vi "Main.vi"() -> ()   [LabVIEW 2025]
doc: "This template is for the Queued Message Handler design pattern.\n\nThe Event Handling Loop generates messages based on user interface actions.\n\nThe Message Handling Loop processes messages generated by the Event Handling Loop, or by other messages. The messages are string values, so new messages can be added easily to the Message Cases case structure in the Message Handling Loop. Each message cluster can also provide an optional value for Message Data, which is a variant that can be converted to whatever message-specific data is required."
uses:
  controls/UI Data.ctl
  support/Message Queue/Enqueue Message (Single).vi
  config/Stop Parse.vi
  <vilib>/Utility/error.llb/Error Cluster From Error Code.vi
  <vilib>/ErrorRing/Error Ring.xnode
  support/Message Queue/Message Queue.lvlib
  support/User Event - Stop/User Event - Stop.lvlib
panel:
  in  "CSV config sections":string[](array[string])=["RAW", "BESTXYZ", "TIME", "PSRDOP", "HWMONITOR", "GPGSV"]
  in  "OEM719 Log Parser":enum32{"OEM719 Log Parser", "Prompt"}(tab)
  in  "Stop Parse Btn":bool
  in  "Start Parse Btn":bool
  out "Notifications":string
  in  "Exit":bool
  in  "OEM 719 Simulated Log":path
  in  "offset (in bytes) (1000000)":i64=1000000
  in  "Duration (s)":dbl=30.0
  out "Elapsed_time":dbl format="%<%H:%M:%S%2u>t"
  in  "CSV File Names":string[](array[string])=["GPS RAW DATA.csv", "BESTXYZ.csv", "GPS TIME.csv", "GPS PSRDOP.csv", "GPS HWMONITOR.csv", "GPS GPGSV.csv"]
  out "Array":path[](array[path])
  # "OEM 719 Log Parser"
  # "Develop a LabVIEW application in a project to parse the provided “OEM719 Simulated Log.txt” data into separate .csv files for each distinct message type.\n•\tThe script should capture data at a frequency of 1 Hz for a duration of 30 seconds. \n•\tParsing the “OEM719 Simulated Log.txt” file should begin from an offset of 1000000 bytes from the start of the file or when the GPS acquires lock.\n•\t Each .csv file should include headers as specified in the OEM719 manual or see “GPS Logs Solution” for reference. \n•\tDo not modify the OEM719 Simulated Log.txt file."
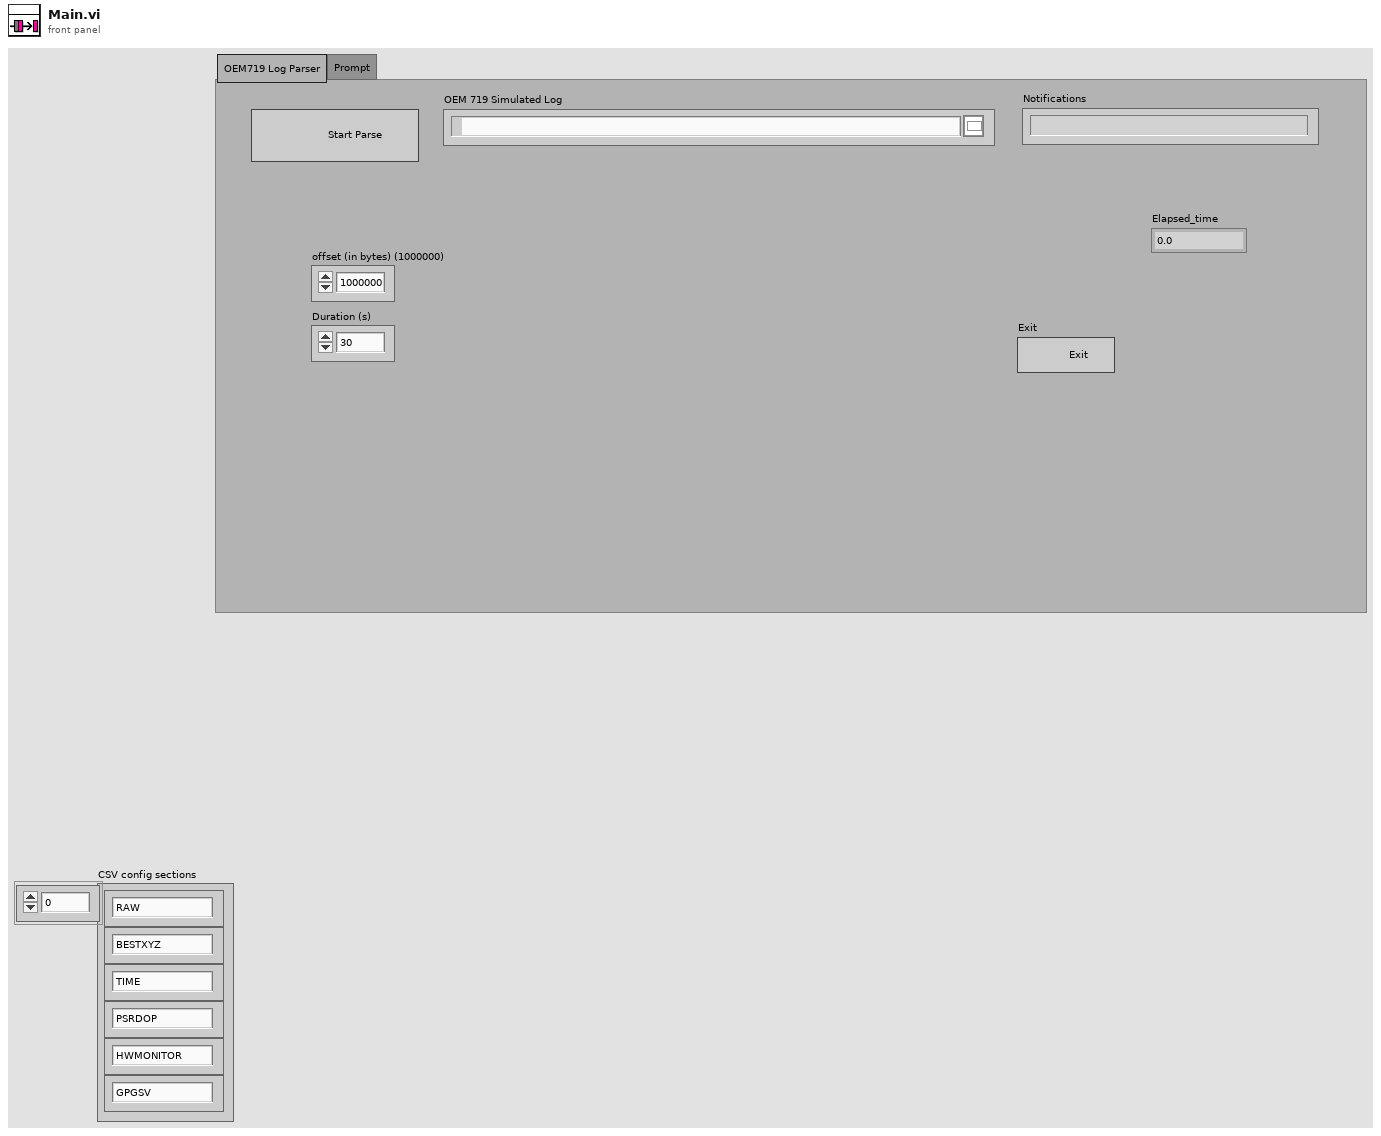
[diagram p1: front panel]
types:
  T1 = typedef "UI Data.ctl" = cluster{"Initialize Btn Ref":refnum<vi>, "Start Parse":refnum<vi>, "Data Display Ref":refnum<vi>, "Exit Button Ref":refnum<vi>}
  T2 = typedef "Message Queue.lvlib/All Message Queues.ctl" = cluster{"UI":refnum<queue>}
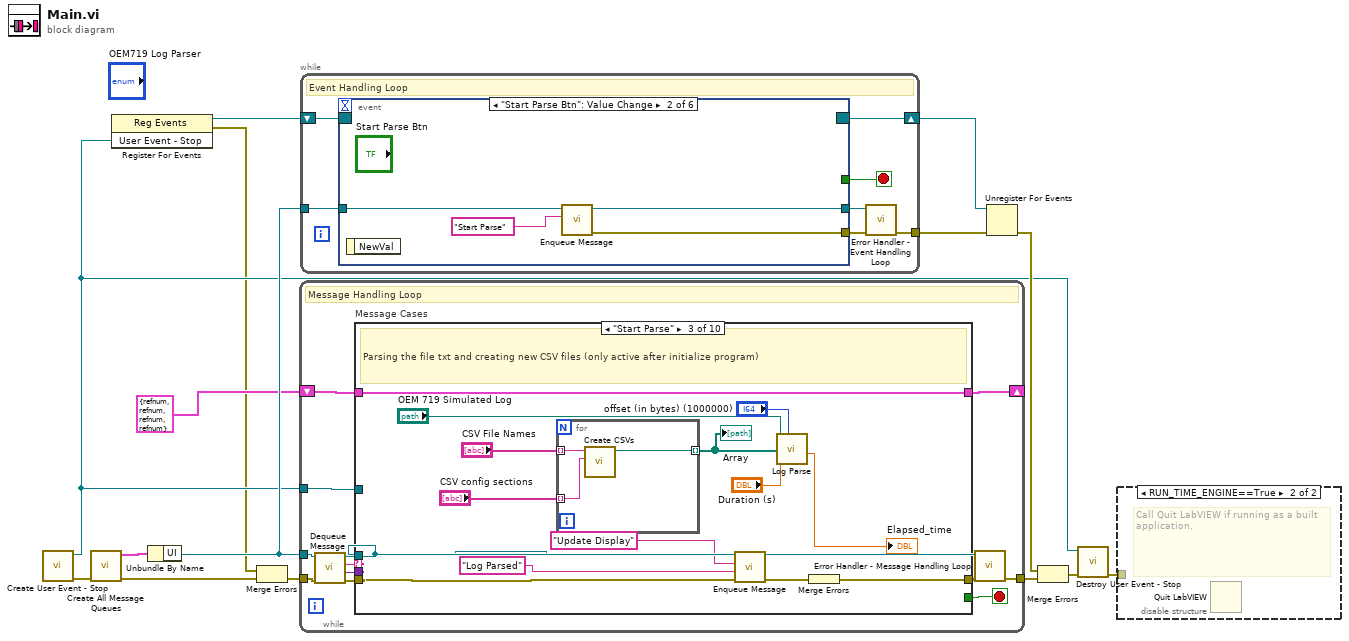
[diagram p0: block diagram]
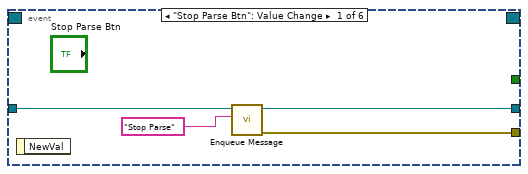
[diagram p3: hidden frame]
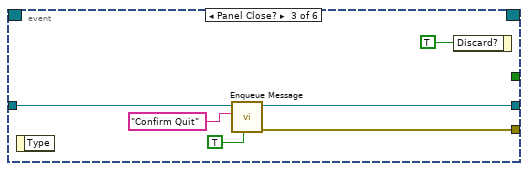
[diagram p4: hidden frame]
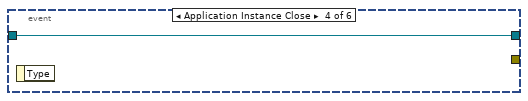
[diagram p5: hidden frame]
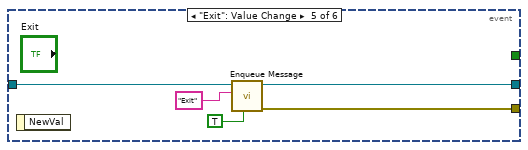
[diagram p6: hidden frame]
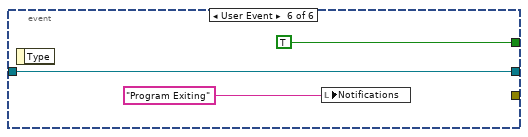
[diagram p7: hidden frame]
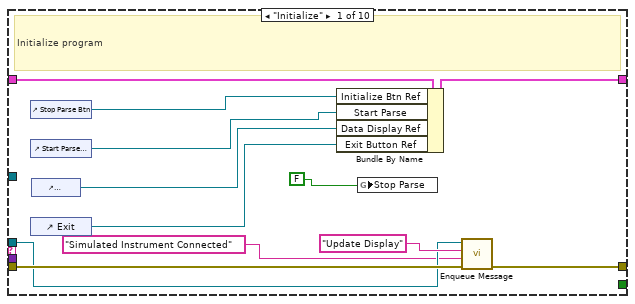
[diagram p8: hidden frame]
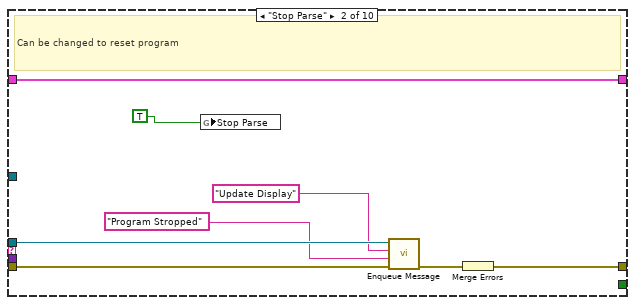
[diagram p9: hidden frame]
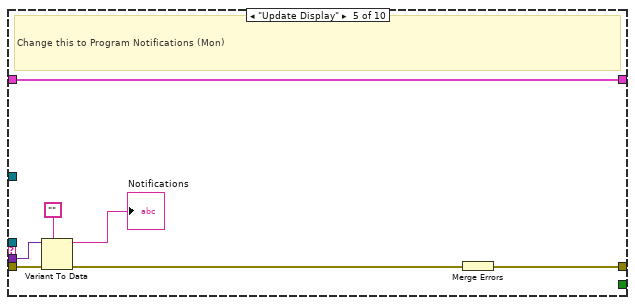
[diagram p11: hidden frame]
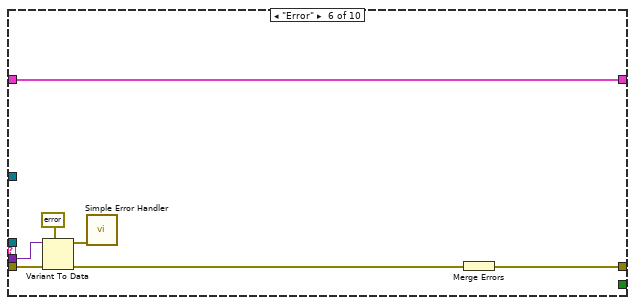
[diagram p12: hidden frame]
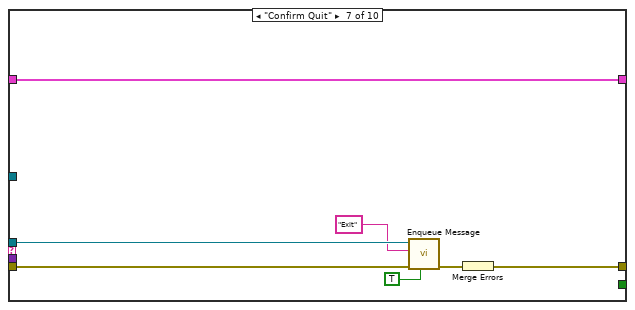
[diagram p13: hidden frame]
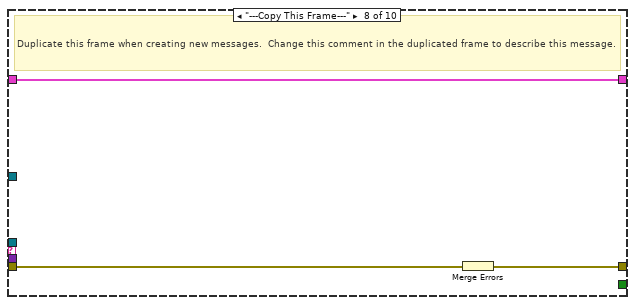
[diagram p14: hidden frame]
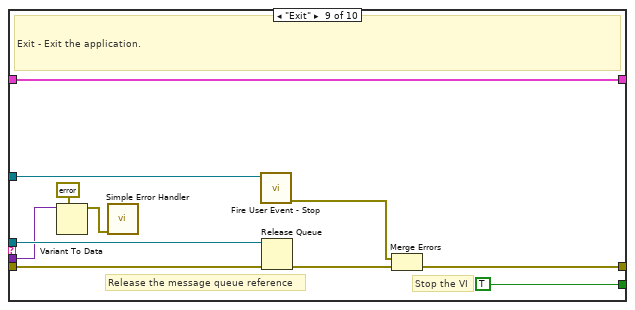
[diagram p15: hidden frame]
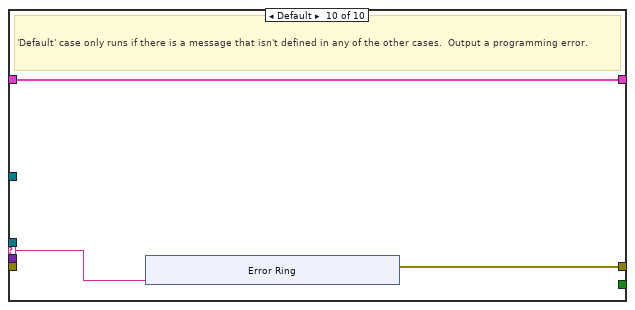
[diagram p16: hidden frame]
diagram:
  n1 = call "Create User Event - Stop.vi"() -> ("error out"=w11:errorcluster, "User Event - Stop"=w3:refnum<user-event>)  [unwired: 10 in]
  n2 = call "Create All Message Queues.vi"("error in (no error)"=w11) -> ("error out"=w15:errorcluster, "Message Queues out"=w14:T2)  [unwired: 9 in]
  n3 = register-events(w3) -> (reference out=w4:refnum<event-registration>, error out=w1:errorcluster)  [unwired: 2 in]
  n4 = Unbundle By Name(w14) -> ("UI"=w12:refnum<queue>)
  n5 = Merge Errors(w1, w15) -> (w2:errorcluster)
  n6 = while {
    tunnel: w12 -> [w19]
    shift-right: [w26] -> _
    shift-left: T1 {"Initialize Btn Ref"=refnum, "Start Parse"=refnum, "Data Display Ref"=refnum, "Exit Button Ref"=refnum} ("Data Cluster") -> [w27]
    tunnel: w3 -> [w24]
    tunnel: w2 -> [w23]
    tunnel: [w17] -> w13
    stop <- w25 stop-if-true
    # "Message Handling Loop"
    n7 = call "Dequeue Message.vi"("error in (no error)"=w23, "Message Queue"=w19) -> ("error out"=w22:errorcluster, "Message Data"=w20:variant, "Message"=w21:string, "dup Message Queue"=w18:refnum<queue>)  [unwired: 6 in]
    n8 = case "Message Cases" shown="\"Start Parse\"" w21 {
      selector: w21 -> [_ _ _ _ _ _ _ _ _ w102]
      tunnel: w18 -> [w31 w43 w50 _ _ _ w83 _ w101 _]
      tunnel: w22 -> [w38 w45 w49 w66 w71 w80 w87 w90 w94 _]
      tunnel: [w39 w46 w60 w66 w72 w74 w85 w88 w97 w103] -> w16
      tunnel: w27 -> [w37 w47 w61 w65 w73 w79 w86 w89 w100 w104]
      tunnel: [w36 w47 w61 w65 w73 w79 w86 w89 w100 w104] -> w26
      tunnel: [_ _ _ _ _ _ _ _ TRUE _] -> w25
      tunnel: w20 -> [_ _ _ _ w70 w78 _ _ w91 _]
      tunnel: w24 -> [_ _ _ _ _ _ _ _ w96 _]
      frame "Initialize" {
        # "Initialize program"
        n9 = control-ref of="Stop Parse Btn"() -> (w35:refnum<vi>)
        n10 = control-ref of="Start Parse Btn"() -> (w29:refnum<vi>)
        n11 = control-ref of="Exit"() -> (w33:refnum<vi>)
        n12 = control-ref of="Notifications"() -> (w34:refnum<vi>)
        n13 = Bundle By Name(cluster=w37, "Initialize Btn Ref"=w35, "Start Parse"=w29, "Data Display Ref"=w34, "Exit Button Ref"=w33) -> (w36:T1)
        n14 = global write "Stop Parse.vi" "Stop Parse"(FALSE) -> ()
        n15 = call-poly "Enqueue Message.vi"("error in (no error)"=w38, "Message Data"="Simulated Instrument Connected" ("Initial Message"), "Message"="Update Display", "Message Queue"=w31) -> ("error out"=w39:errorcluster)  [unwired: 6 in, 1 out]
      }
      frame "Stop Parse" {
        # "Can be changed to reset program"
        n16 = global write "Stop Parse.vi" "Stop Parse"(TRUE) -> ()
        n17 = call-poly "Enqueue Message.vi"("error in (no error)"=w45, "Message Data"="Program Stropped" ("\"Do Something\" button pressed"), "Message"="Update Display", "Message Queue"=w43) -> ("error out"=w44:errorcluster)  [unwired: 6 in, 1 out]
        n18 = Merge Errors(w44) -> (w46:errorcluster)
      }
      frame "Start Parse" {
        # "Parsing the file txt and creating new CSV files (only active after initialize program)"
        n19 = for {
          tunnel: "CSV File Names" -> [w64] mode=indexing
          tunnel: "CSV config sections" -> [w63] mode=indexing
          tunnel: [w62] -> w54 mode=indexing
          n20 = call "Create CSVs.vi"("CSV config section"=w63, "CSV File Name"=w64) -> ("CSV refnum"=w62:path)  [unwired: 8 in, 1 out]
        }
        "Array" <- w54
        n21 = call-poly "Enqueue Message.vi"("error in (no error)"=w49, "Message Data"="Log Parsed" ("\"Do Something Else\" button pressed"), "Message"="Update Display", "Message Queue"=w50) -> ("error out"=w59:errorcluster)  [unwired: 6 in, 1 out]
        n22 = call "Log Parse.vi"("offset (in bytes) (1000000)"="offset (in bytes) (1000000)", "Duration"="Duration (s)", "CSV Refnum Files"=w54, "OEM 719 Simulated Log"="OEM 719 Simulated Log") -> ("Elapsed_time"=→"Elapsed_time":dbl)  [unwired: 7 in]
        n23 = Merge Errors(w59) -> (w60:errorcluster)
      }
      frame "Edit Parser" {
        # "To DO: (no time)\nSplit Start Parse into create CSV and Log Parse msgs\nFinish Stop Parse"
        # "Should be able to change the sampling rate freq HZ, time and offset bytes/GPS Locks"
      }
      frame "Update Display" {
        # "Change this to Program Notifications (Mon)"
        n24 = Variant To Data(error in=w71, type="", Variant=w70) -> (data=→"Notifications":string, error out=w68:errorcluster)
        n25 = Merge Errors(w68) -> (w72:errorcluster)
      }
      frame "Error" {
        n26 = Variant To Data(error in=w80, type=errorcluster {"status"=FALSE, "code"=0, "source"=""} ("error constant"), Variant=w78) -> (data=w76:errorcluster, error out=w75:errorcluster)
        n27 = call <vilib>:"Simple Error Handler.vi"("error in (no error)"=w76) -> ()  [unwired: 4 in, 5 out]
        n28 = Merge Errors(w75) -> (w74:errorcluster)
      }
      frame "Confirm Quit" {
        n29 = call-poly "Enqueue Message.vi"("Priority Message? (F)"=TRUE, "error in (no error)"=w87, "Message"="Exit", "Message Queue"=w83) -> ("error out"=w84:errorcluster)  [unwired: 6 in, 1 out]
        n30 = Merge Errors(w84) -> (w85:errorcluster)
      }
      frame "---Copy This Frame---" {
        # "Duplicate this frame when creating new messages.  Change this comment in the duplicated frame to describe this message."
        n31 = Merge Errors(w90) -> (w88:errorcluster)
      }
      frame "Exit" {
        # "Stop the VI"
        # "Release the message queue reference"
        # "Exit - Exit the application."
        n32 = Variant To Data(type=errorcluster {"status"=FALSE, "code"=0, "source"=""} ("error constant"), Variant=w91) -> (data=w92:errorcluster)  [unwired: 1 in, 1 out]
        n33 = call <vilib>:"Simple Error Handler.vi"("error in (no error)"=w92) -> ()  [unwired: 4 in, 5 out]
        n34 = call "Fire User Event - Stop.vi"("User Event - Stop"=w96) -> ("error out"=w95:errorcluster)  [unwired: 10 in]
        n35 = Release Queue(queue=w101, error in (no error)=w94) -> (error out=w98:errorcluster)  [unwired: 1 in, 2 out]
        n36 = Merge Errors(w95, w98) -> (w97:errorcluster)
      }
      frame Default {
        # "'Default' case only runs if there is a message that isn't defined in any of the other cases.  Output a programming error."
        n37 = xnode "Error Ring"("parameter 0"=w102) -> ("error out"=w103:errorcluster)
      }
    }
    n38 = call "Error Handler - Message Handling Loop.vi"("error in (no error)"=w16, "Message Queue"=w18) -> ("dup error in"=w17:errorcluster)  [unwired: 8 in, 1 out]
  }
  n39 = while {
    tunnel: w12 -> [w118]
    shift-right: [w116] -> w8
    shift-left: w4 -> [w117]
    tunnel: [w112] -> w5
    stop <- w114 stop-if-true
    # "Event Handling Loop"
    n40 = event shown="[1] \"Start Parse Btn\": Value Change" {
      selector: w117 -> [_ _ _ _ _ _]
      dyn-events: [_ _ _ _ _ _] -> w116
      timeout: _ -> [_ _ _ _ _ _]
      tunnel: [_ _ _ _ _ TRUE ("Discard?")] -> w114
      tunnel: w118 -> [w122 w126 w131 w133 w138 w141]
      tunnel: [w119 w123 w130 _ w137 _] -> w115
      tunnel: [w121 w125 w129 w133 w136 w141] -> w113
      event "Stop Parse Btn": Value Change {
        n41 = event-data() -> ()  [unwired: 1 in, 1 out]
        n42 = call-poly "Enqueue Message.vi"("Message"="Stop Parse", "Message Queue"=w122) -> ("error out"=w119:errorcluster, "dup Message Queue"=w121:refnum<queue>)  [unwired: 8 in]
      }
      event "Start Parse Btn": Value Change {
        n43 = event-data() -> ()  [unwired: 1 in, 1 out]
        n44 = call-poly "Enqueue Message.vi"("Message"="Start Parse", "Message Queue"=w126) -> ("error out"=w123:errorcluster, "dup Message Queue"=w125:refnum<queue>)  [unwired: 8 in]
      }
      event Panel Close? {
        n45 = event-data() -> ()  [unwired: 1 in, 1 out]
        n46 = call-poly "Enqueue Message.vi"("Priority Message? (F)"=TRUE, "Message"="Confirm Quit", "Message Queue"=w131) -> ("error out"=w130:errorcluster, "dup Message Queue"=w129:refnum<queue>)  [unwired: 7 in]
        n47 = event-data("Discard?"=TRUE) -> ()  [unwired: 1 in, 1 out]
      }
      event Application Instance Close {
        n48 = event-data() -> ()  [unwired: 1 in, 1 out]
      }
      event "Exit": Value Change {
        n49 = event-data() -> ()  [unwired: 1 in, 1 out]
        n50 = call-poly "Enqueue Message.vi"("Priority Message? (F)"=TRUE, "Message"="Exit", "Message Queue"=w138) -> ("error out"=w137:errorcluster, "dup Message Queue"=w136:refnum<queue>)  [unwired: 7 in]
      }
      event User Event {
        n51 = event-data() -> ()  [unwired: 1 in, 1 out]
        n52 = local write "Notifications"("Program Exiting" ("VI Stopped")) -> ()
      }
    }
    n53 = call "Error Handler - Event Handling Loop.vi"("error in (no error)"=w115, "Message Queue"=w113) -> ("dup error in"=w112:errorcluster)  [unwired: 8 in, 1 out]
  }
  n54 = Unregister For Events(event registration refnum=w8, error in=w5) -> (error out=w9:errorcluster)
  n55 = Merge Errors(w9, w13) -> (w10:errorcluster)
  n56 = call "Destroy User Event - Stop.vi"("error in (no error)"=w10, "User Event - Stop"=w3) -> ("error out"=w6:errorcluster)  [unwired: 9 in]
  n57 = disable-structure shown="RUN_TIME_ENGINE==True" {
    disable-tunnel: w6 -> [_ _]
    frame condition #0 (active) {
    }
    frame condition #1 {
      # "Call Quit LabVIEW if running as a built application."
      n58 = Quit LabVIEW() -> ()  [unwired: 1 in]
    }
  }
